vi "Start Stream.vi"(8 "error in (no error)":errorcluster, 11 "Ni-Scope Digitizer in":refnum<class "Ni-Scope Digitizer.lvclass">) -> (0 "error out":errorcluster, 3 "Ni-Scope Digitizer out":refnum<class "Ni-Scope Digitizer.lvclass">)   [LabVIEW 2016, in "Ni-Scope Digitizer.lvclass"]
uses:
  Ni-Scope Digitizer.lvclass
  C:/github/NHMFL_Core/Libraries/Instruments/Pulse Driver/Pulse Driver.lvclass
  Instruments/Pulse Driver/Pulse Driver.lvclass/Pulse Driver.ctl
  Ni-Scope Digitizer.lvclass/Ni-Scope Digitizer.ctl
  Instruments/Pulse Driver/Read Binary sample width.vi
  <instrlib>/niScope/Acquire/Fetch/niScope Multi Fetch Binary 16.vi
  <instrlib>/niScope/Acquire/Fetch/niScope Multi Fetch Binary 32.vi
  Instruments/Pulse Driver/Pulse Driver.lvclass
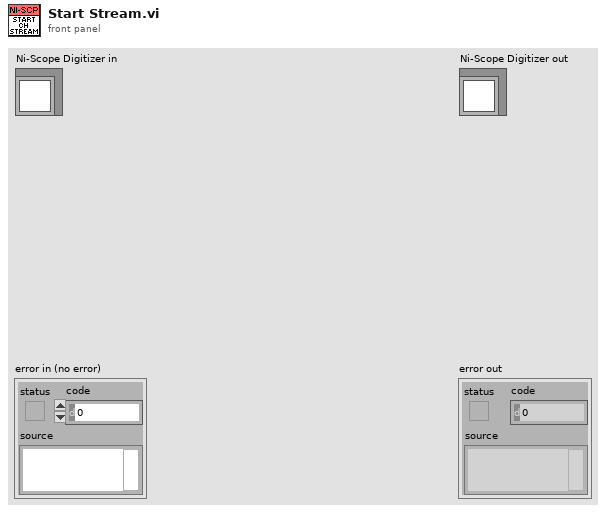
[diagram p1: front panel]
types:
  T1 = typedef "Pusle Driver Configuration.ctl" = cluster{"Pre-trigger duration":dbl, "Post-trigger duration":dbl, "Rate":dbl, "Ranges":dbl[], "Re-name channels":string[], "Active channels":string, "External clock":bool}
  T2 = cluster{"actualSamples":i32, "absoluteInitialX":dbl, "relativeInitialX":dbl, "xIncrement":dbl, "offset":dbl, "gain":dbl, "reserved1":dbl, "reserved2":dbl}[]
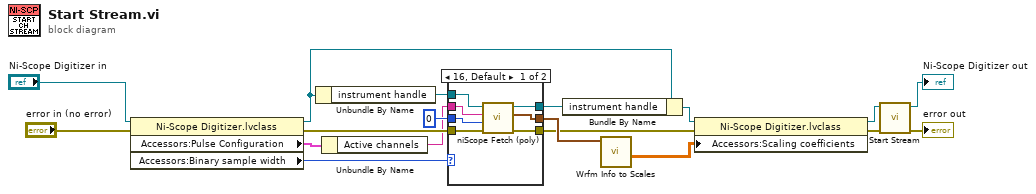
[diagram p0: block diagram]
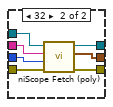
[diagram p2: hidden frame]
diagram:
  n1 = property class="Ni-Scope Digitizer.lvclass"(reference="Ni-Scope Digitizer in", error in="error in (no error)") -> (reference out=w2:refnum<class "Ni-Scope Digitizer.lvclass">, error out=w13:errorcluster, "Accessors:Pulse Configuration"=w10:T1, "Accessors:Binary sample width"=w9:i32)
  n2 = Unbundle By Name(w2) -> ("instrument handle"=w16:refnum<k15>)
  n3 = Unbundle By Name(w10) -> ("Active channels"=w11:string)
  n4 = case shown="16, Default" w9 {
    tunnel: w11 -> [w25 w32]
    tunnel: w16 -> [w24 w31]
    tunnel: w13 -> [w23 w30]
    tunnel: [w22 w29] -> w7
    tunnel: [w21 w28] -> w8
    tunnel: [w20 w27] -> w1
    tunnel: 0 ("Accessors:Samples per read") -> [w19 w26]
    frame 16, Default {
      n5 = call-poly <instrlib>:"niScope Fetch (poly).vi"("error in"=w23, "numSamples"=w19, "channels"=w25, "instrument handle"=w24) -> ("error out"=w22:errorcluster, "wfm info"=w21:T2, "instrument handle out"=w20:refnum<k15>)  [unwired: 4 in, 1 out]
    }
    frame 32 {
      n6 = call-poly <instrlib>:"niScope Fetch (poly).vi"("error in"=w30, "numSamples"=w26, "channels"=w32, "instrument handle"=w31) -> ("error out"=w29:errorcluster, "wfm info"=w28:T2, "instrument handle out"=w27:refnum<k15>)  [unwired: 4 in, 1 out]
    }
  }
  n7 = Bundle By Name(cluster=w2, "instrument handle"=w1) -> (w3:refnum<class "Ni-Scope Digitizer.lvclass">)
  n8 = call "Wrfm Info to Scales.vi"("wfm info"=w8) -> ("Scaling coefficients"=w6:dbl[][])  [unwired: 8 in, 2 out]
  n9 = property class="Ni-Scope Digitizer.lvclass"(reference=w3, error in=w7, "Accessors:Scaling coefficients"=w6) -> (reference out=w4:refnum<class "Ni-Scope Digitizer.lvclass">, error out=w5:errorcluster)
  n10 = call-parent "Start Stream.vi"("error in (no error)"=w5, "Pulse Driver in"=w4) -> ("error out"=→"error out":errorcluster, "Pulse Driver out"=→"Ni-Scope Digitizer out":refnum<class "Ni-Scope Digitizer.lvclass">)  [unwired: 8 in]
